vi "SetChannelConf-OutSession.vi"(8 "error in":errorcluster, 9 "Out Session":refnum<k21>, 10 "Channel Num":u32, 11 "CAN-NI":refnum<class "CAN-NI.lvclass">) -> (0 "error out":errorcluster, 3 "CAN-NI":refnum<class "CAN-NI.lvclass">)   [LabVIEW 2019, in "CAN-NI.lvlib" / "CAN-NI.lvclass"]
uses:
  CAN-NI.lvclass
  TypeDef/ChannelProperty.ctl
  CAN-Interface/TypeDef/Def-Termination.ctl
  CAN-Interface/TypeDef/Def-Transmit Mode.ctl
  CAN-Interface/TypeDef/Def-Protocol.ctl
  CAN-NI.lvclass/CAN-NI.ctl
  CAN-Interface/Class-Interface.lvclass
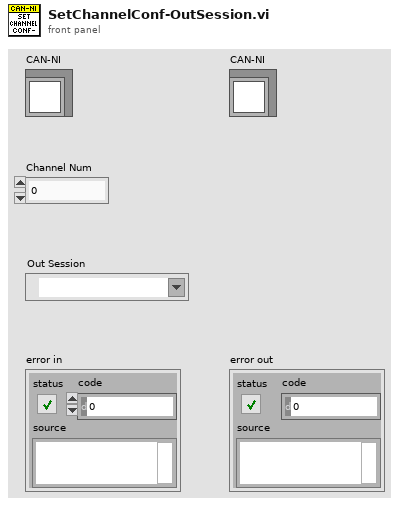
[diagram p1: front panel]
types:
  T1 = typedef "CAN-NI.lvlib/CAN-NI.lvclass/ChannelProperty.ctl" = cluster{"CAN-cluster":refnum<k21>, "CAN-Frames":refnum<k21>[], "Termination":T2, "Transmit Mode":T3, "Frame Out Session":refnum<k21>, "Frame In Session":refnum<k21>, "Protocol":T4}
  T2 = typedef "CAN-Interface.lvlib/Class-Interface.lvclass/Def-Termination.ctl" = enum8{"on", "off"}
  T3 = typedef "CAN-Interface.lvlib/Class-Interface.lvclass/Def-Transmit Mode.ctl" = enum16{"Queued", "Stream"}
  T4 = typedef "CAN-Interface.lvlib/Class-Interface.lvclass/Def-Protocol.ctl" = enum16{"CAN", "CAN FD"}
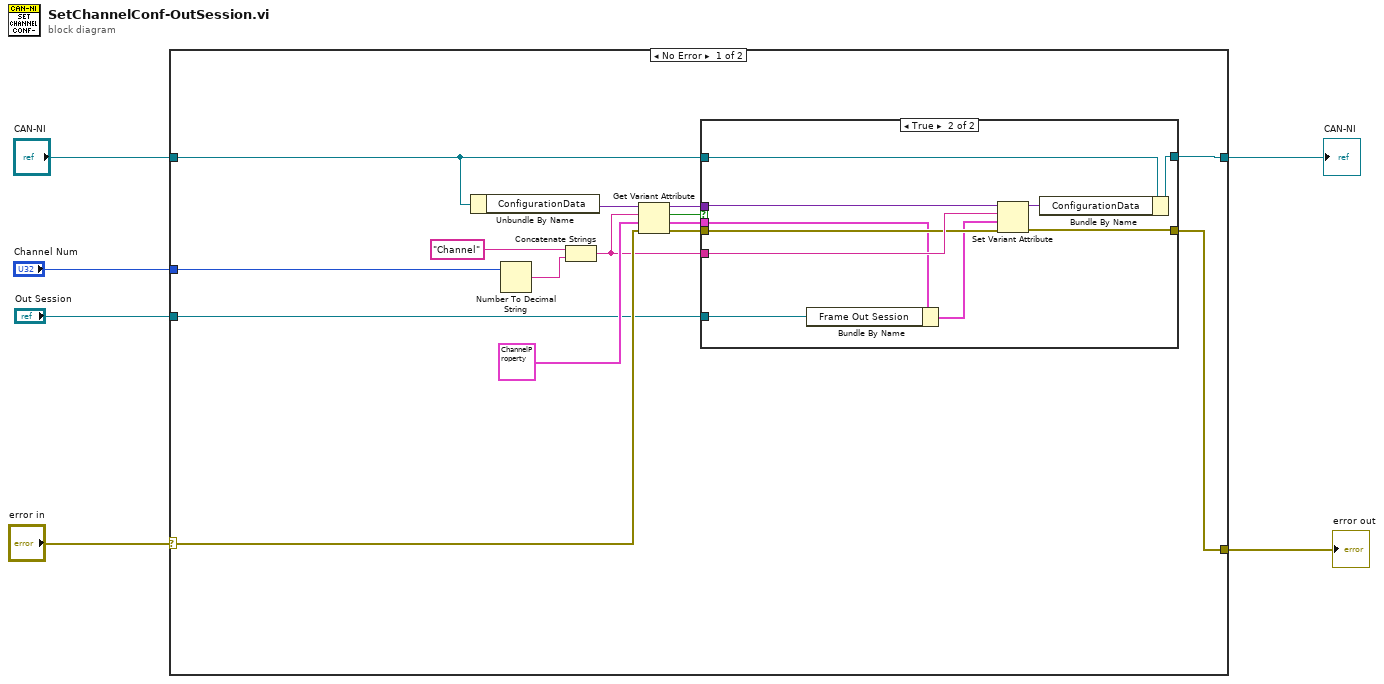
[diagram p0: block diagram]
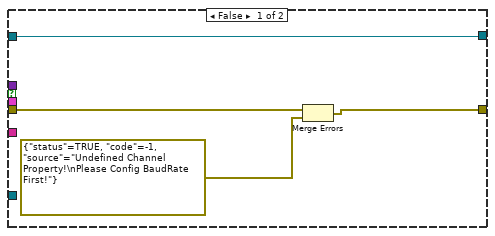
[diagram p2: hidden frame]
diagram:
  n1 = case shown="No Error" "error in" {
    selector: "error in" -> [w14 w37]
    tunnel: "CAN-NI" -> [w9 w36]
    tunnel: "Channel Num" -> [w19 _]
    tunnel: [w12 w37] -> w3
    tunnel: [w8 w36] -> w2
    tunnel: "Out Session" -> [w7 _]
    frame No Error {
      n2 = Unbundle By Name(w9) -> ("ConfigurationData"=w18:variant)
      n3 = Number To Decimal String(number=w19) -> (decimal integer string=w21:string)  [unwired: 1 in]
      n4 = Concatenate Strings("Channel" ("string"), w21) -> (w10:string)
      n5 = Get Variant Attribute(Variant=w18, name=w10, default value (empty Variant)=T1 {"CAN-cluster"="", "CAN-Frames"=[], "Termination"=enum."on", "Transmit Mode"=enum."Queued", "Frame Out Session"="", "Frame In Session"="", "Protocol"=enum."CAN"} ("ChannelProperty"), error in=w14) -> (duplicate Variant=w11:variant, found=w16:bool, value=w15:T1, error out=w13:errorcluster)
      n6 = case shown="True" w16 {
        tunnel: w15 -> [_ w28]
        tunnel: w13 -> [w25 w32]
        tunnel: [w23 w33] -> w12
        tunnel: w11 -> [_ w35]
        tunnel: w10 -> [_ w34]
        tunnel: w9 -> [w22 w31]
        tunnel: [w22 w29] -> w8
        tunnel: w7 -> [_ w26]
        frame False {
          n7 = Merge Errors(w25, errorcluster {"status"=TRUE, "code"=-1, "source"="Undefined Channel Property!\nPlease Config BaudRate First!"} ("error in (no error)")) -> (w23:errorcluster)
        }
        frame True {
          n8 = Bundle By Name(cluster=w28, "Frame Out Session"=w26) -> (w27:T1)
          n9 = Set Variant Attribute(Variant=w35, name=w34, value=w27, error in=w32) -> (Variant out=w30:variant, error out=w33:errorcluster)  [unwired: 1 out]
          n10 = Bundle By Name(cluster=w31, "ConfigurationData"=w30) -> (w29:refnum<class "CAN-NI.lvclass">)
        }
      }
    }
    frame Error {
    }
  }
  "error out" <- w3
  "CAN-NI" <- w2
